vi "SRV_PM_Packet Mode Enable.vi"(6 "Packet Mode Enable (T)":bool=TRUE, 8 "error in (no error)":errorcluster, 11 "connection ID":refnum<k5>) -> (0 "error out":errorcluster, 3 "connection ID out":refnum<k5>)   [LabVIEW 2009]
panel:
  out "Command Sent":string
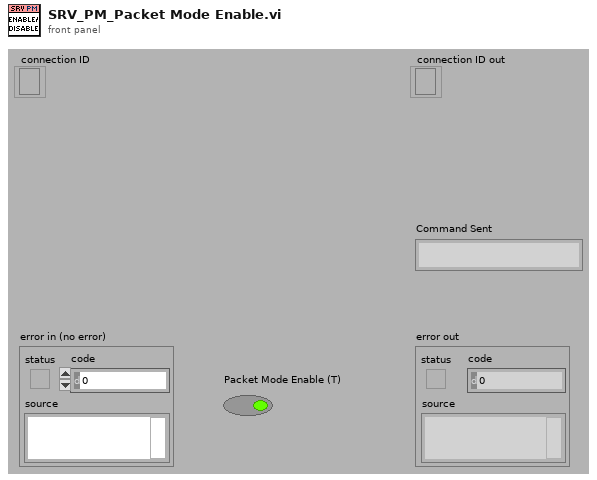
[diagram p1: front panel]
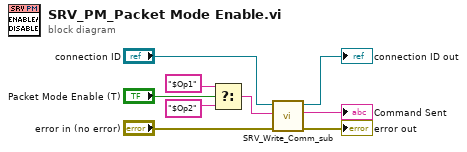
[diagram p0: block diagram]
diagram:
  n1 = Select(t="$Op1", s="Packet Mode Enable (T)", f="$Op2") -> (s? t:f=w2:string)
  n2 = call "SRV_Write_Comm_sub.vi"("error in (no error)"="error in (no error)", "Command Sent"=w2, "SRV In"="connection ID") -> ("error out"=→"error out":errorcluster, "Command Sent dup"=→"Command Sent":string, "SRV Out"=→"connection ID out":refnum<k5>)  [unwired: 6 in]
